vi "Format Ranges.vi"(10 "Ranges Array":sgl[](array[numeric])) -> (2 "Ranges":T1)   [LabVIEW 2020, in "FormulaG.lvlib" / "FormulaG API.lvclass"]
uses:
  FormulaG API.lvclass
  FormulaG-Common/Ranges.ctl
  FormulaG API.lvclass/FormulaG API.ctl
  FormulaG-Common/FormulaG-Common.lvlib
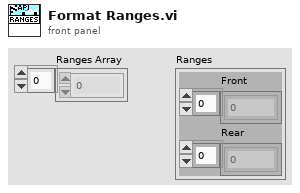
[diagram p1: front panel]
types:
  T1 = typedef "FormulaG-Common.lvlib/Ranges.ctl" = cluster{"Front":sgl[], "Rear":sgl[]}
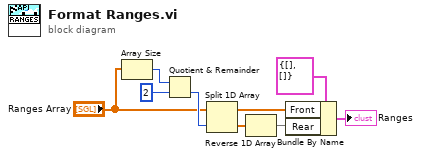
[diagram p0: block diagram]
diagram:
  n1 = Array Size(array="Ranges Array") -> (size(s)=w9:i32)
  n2 = Quotient & Remainder(x=w9, y=2) -> (floor(x/y)=w7:i32)  [unwired: 1 out]
  n3 = Split 1D Array(array="Ranges Array", index=w7) -> (first subarray=w4:sgl[], second subarray=w5:sgl[])
  n4 = Reverse 1D Array(array=w5) -> (reversed array=w3:sgl[])
  n5 = Bundle By Name(cluster=T1 {"Front"=[], "Rear"=[]} ("Ranges"), "Front"=w4, "Rear"=w3) -> (→"Ranges":T1)
